vi "Read Set.vi"(8 "error in (no error)":errorcluster, 11 "Option in":refnum<class "Option.lvclass">) -> (0 "error out":errorcluster, 2 "Set":bool, 3 "Option out":refnum<class "Option.lvclass">)   [LabVIEW 2011, in "Option Parser.lvlib" / "Option.lvclass"]
uses:
  Option.lvclass
  Option.lvclass/Option.ctl
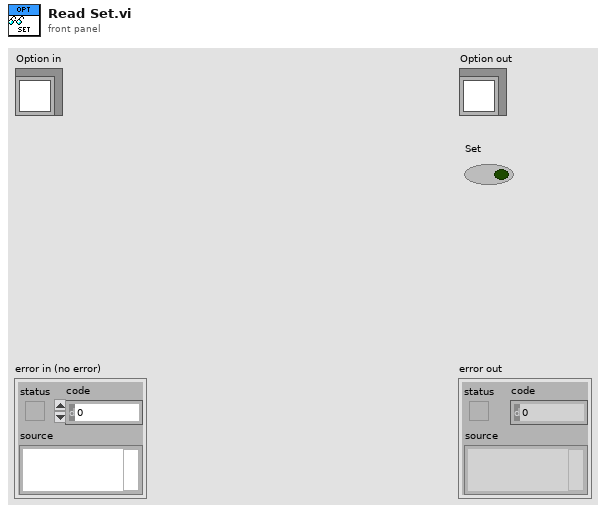
[diagram p1: front panel]
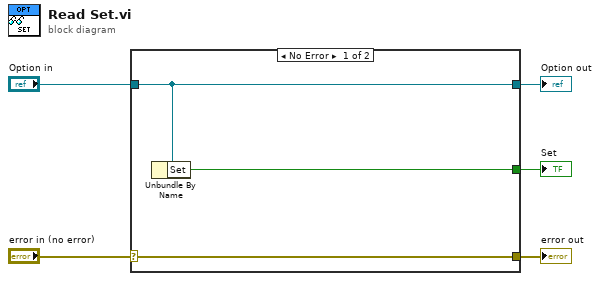
[diagram p0: block diagram]
diagram:
  n1 = case shown="No Error" "error in (no error)" {
    selector: "error in (no error)" -> [w8 w9]
    tunnel: [w8 w9] -> w4
    tunnel: [w7 w10] -> w2
    tunnel: "Option in" -> [w7 w10]
    tunnel: [w6 _] -> w1
    frame No Error {
      n2 = Unbundle By Name(w7) -> ("Set"=w6:bool)
    }
    frame Error {
    }
  }
  "error out" <- w4
  "Option out" <- w2
  "Set" <- w1
